vi "Scripting_G1DeleteToG3Delete.vi"(0 "VI Refnum":refnum<vi>, 1 "SearchVI":path=path "C:/classes/MainVI/MyGoop2/utils/MyGoop2_New.vi", 2 "Get":path=path "C:/classes/MainVI/MyGoop2/utils/MyGoop2_GetAttributesToModify.vi", 5 "error IO":errorcluster) -> (19 "error out":errorcluster)   [LabVIEW 2014]
uses:
  <vilib>/Utility/miscctls.llb/LVPositionTypeDef.ctl
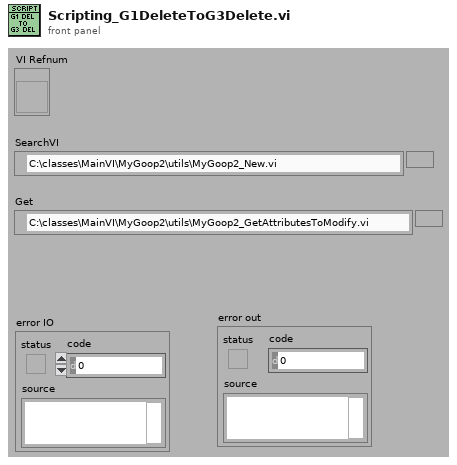
[diagram p1: front panel]
types:
  T1 = cluster{"Delete":refnum<vi>, "GetRef":refnum<vi>, "Block Diagram":refnum<vi>, "MergerErrors":refnum<vi>}
  T2 = typedef "LVPositionTypeDef.ctl" = cluster{"Left":i32, "Top":i32}
  T3 = typedef "LVRectTypeDef.ctl" = cluster{"Left":i16, "Top":i16, "Right":i16, "Bottom":i16}
  T4 = enum16{"Invalid Wire Rule", "Required", "Recommended", "Optional", "Dynamic Dispatch"}
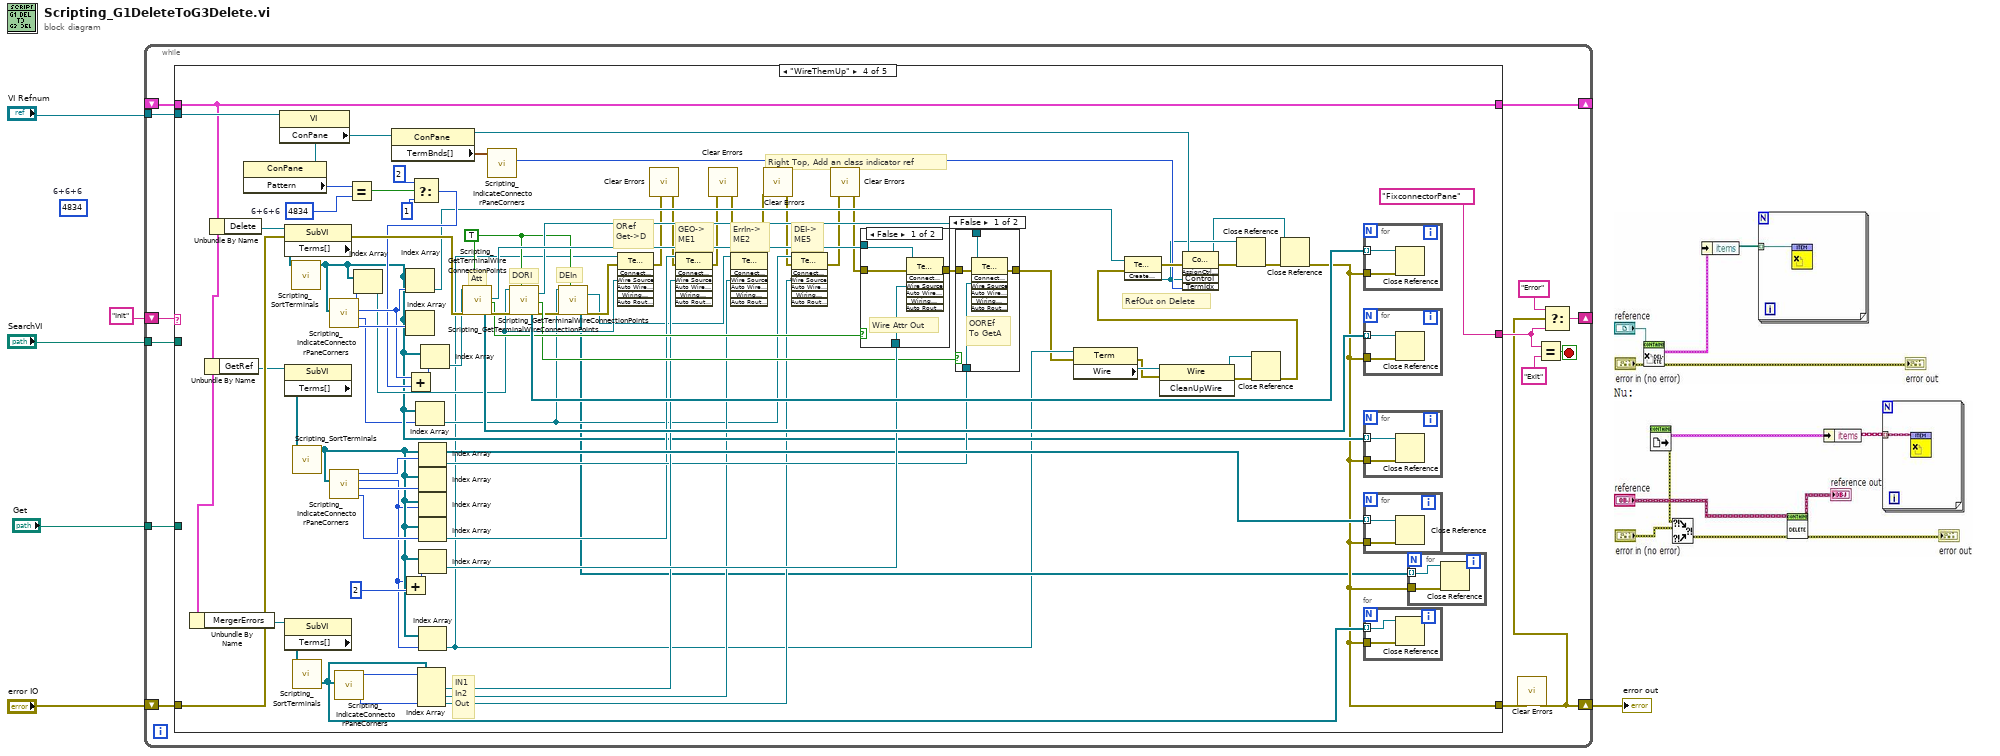
[diagram p0: block diagram]
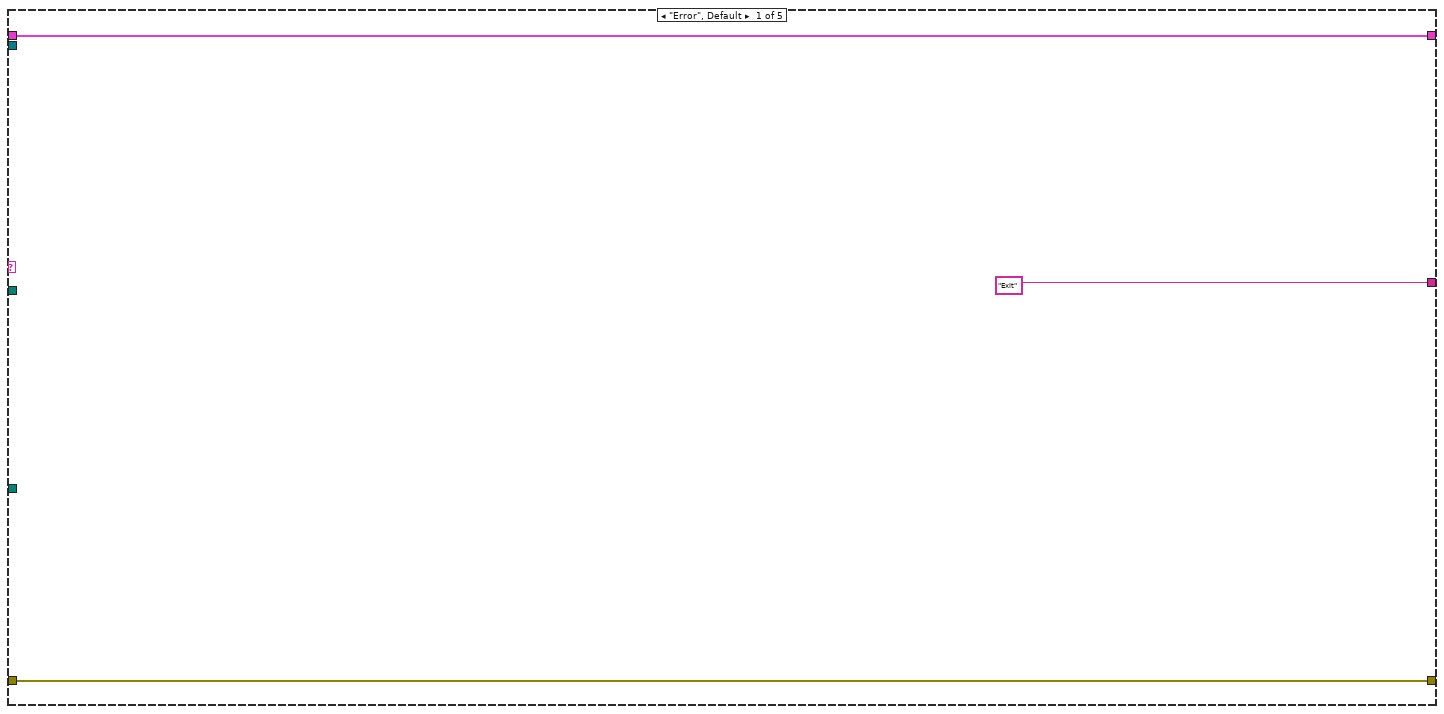
[diagram p2: hidden frame]
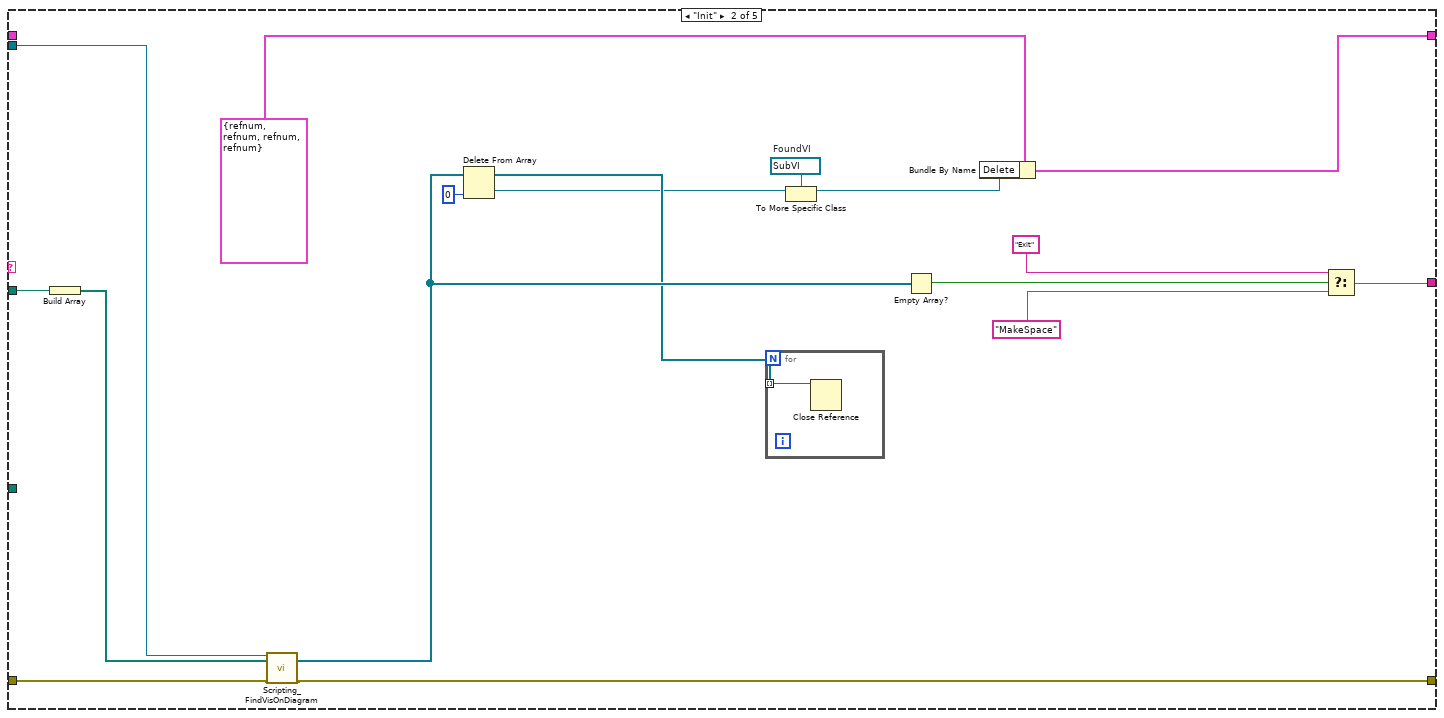
[diagram p3: hidden frame]
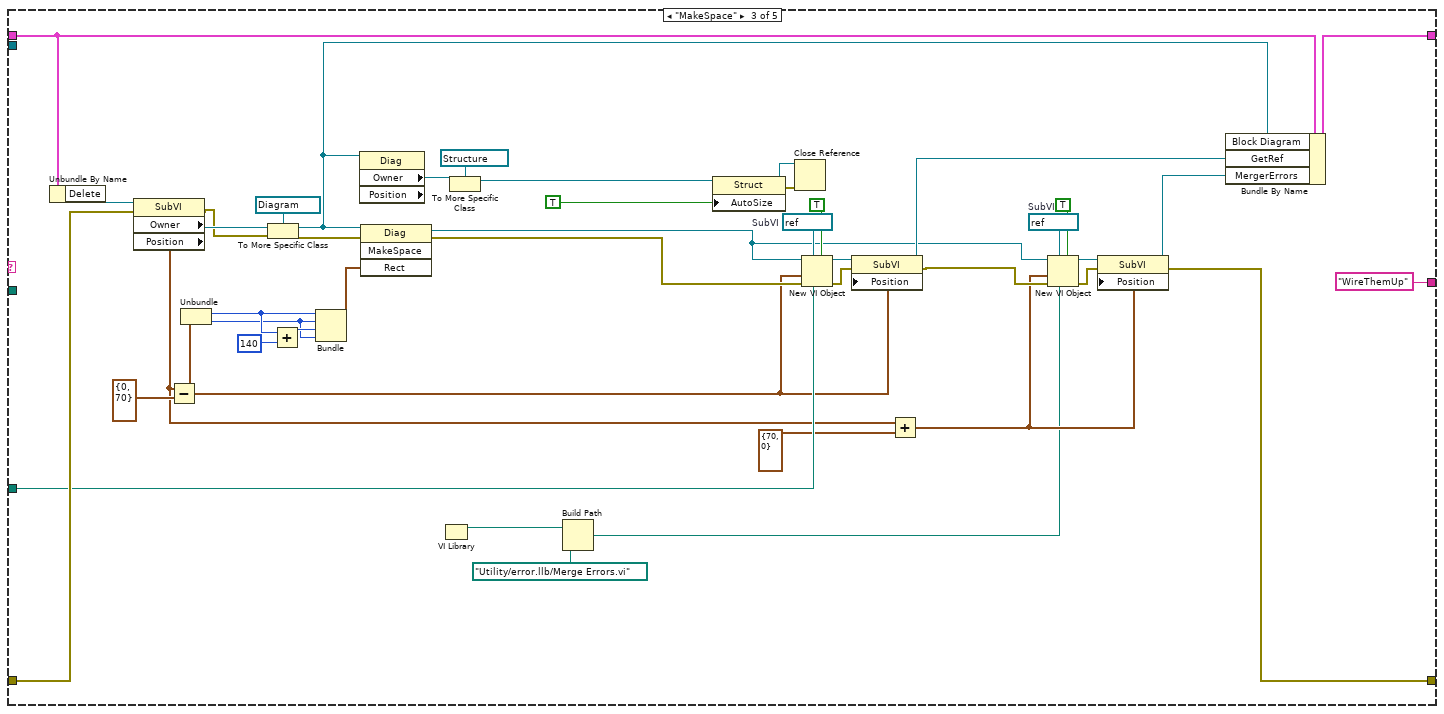
[diagram p4: hidden frame]
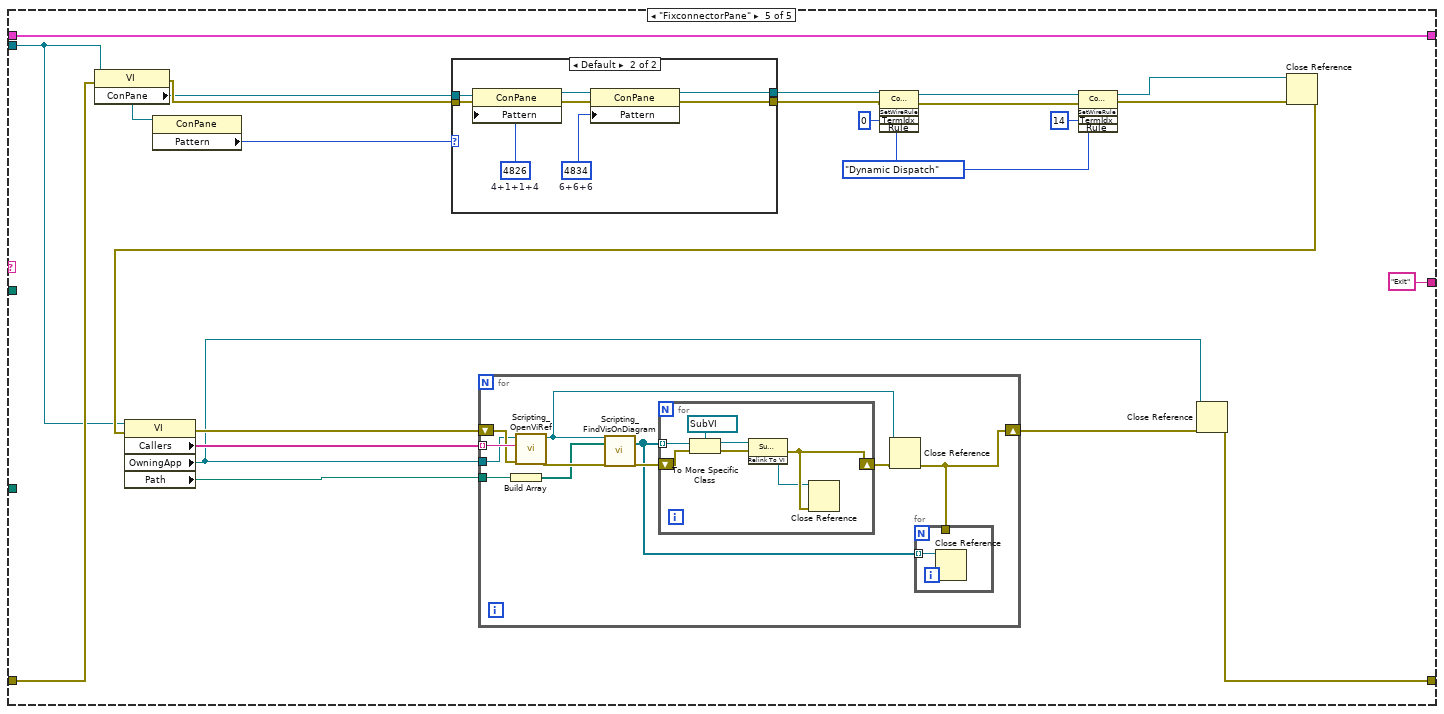
[diagram p7: hidden frame]
diagram:
  (unwired) u32 4834  # 6+6+6
  n1 = while {
    shift-right: [w7] -> w4
    shift-left: "error IO" -> [w20]
    shift-right: [w18] -> _
    shift-left: "Init" -> [w19]
    shift-right: [w13] -> _
    shift-left: _ -> [w12]
    tunnel: "VI Refnum" -> [w11]
    tunnel: "SearchVI" -> [w10]
    tunnel: "Get" -> [w9]
    stop <- w17 stop-if-true
    n2 = case shown="\"WireThemUp\"" w19 {
      tunnel: w20 -> [w23 w38 w84 w165 w210]
      tunnel: [w23 w37 w51 w102 w200] -> w8
      tunnel: ["Exit" w32 "WireThemUp" "FixconnectorPane" "Exit"] -> w14
      tunnel: [w21 w39 w62 w120 w209] -> w13
      tunnel: w12 -> [w21 _ w63 w120 w209]
      tunnel: w11 -> [_ w36 _ w132 w201]
      tunnel: w10 -> [_ w29 _ _ _]
      tunnel: w9 -> [_ _ w77 _ _]
      frame "Error", Default {
      }
      frame "Init" {
        w25 = refnum<vi> refnum  # FoundVI
        n3 = Build Array(w29) -> (w28:path[])
        n4 = call <resource>:"Scripting_FindVisOnDiagram.vi"("ViRef"=w36, "VIsToSerachFor/ViName"=w28, "error in (no error)"=w38) -> ("VisFound"=w31:refnum<vi>[], "error out"=w37:errorcluster)  [unwired: 15 in]
        n5 = Delete From Array(array=w31, index=0) -> (deleted portion=w26:refnum<vi>, array with subset deleted=w27:refnum<vi>[])  [unwired: 1 in]
        n6 = for {
          tunnel: w27 -> [w41] mode=indexing
          n7 = Close Reference(reference=w41) -> ()  [unwired: 1 in, 1 out]
        }
        n8 = To More Specific Class(target class=w25, reference=w26) -> (specific class reference=w24:refnum<vi>)  [unwired: 1 in, 1 out]
        n9 = Empty Array?(array=w31) -> (empty?=w35:bool)
        n10 = Bundle By Name(cluster=T1 {"Delete"=refnum, "GetRef"=refnum, "Block Diagram"=refnum, "MergerErrors"=refnum}, "Delete"=w24) -> (w39:T1)
        n11 = Select(t="Exit", s=w35, f="MakeSpace") -> (s? t:f=w32:string)
      }
      frame "MakeSpace" {
        w53 = refnum<vi> refnum  # SubVI
        w80 = refnum<vi> refnum  # SubVI
        n12 = Unbundle By Name(w63) -> ("Delete"=w85:refnum<vi>)
        n13 = property class="SubVI"(reference=w85, error in=w84) -> (error out=w81:errorcluster, "Owner"=w82:refnum<vi>, "Position"=w42:T2)  [unwired: 1 out]
        n14 = Subtract(x=w42, y=T2 {"Left"=0, "Top"=70}) -> (x-y=w50:T2)
        n15 = Unbundle(w50) -> ("Left"=w73:i32, "Top"=w70:i32)
        n16 = To More Specific Class(target class=refnum<vi> refnum ("Block Diagram"), reference=w82, error in=w81) -> (specific class reference=w58:refnum<vi>, error out=w67:errorcluster)
        n17 = Add(x=w73, y=i16 140 ("Right")) -> (x+y=w71:i32)
        n18 = Bundle("Left"=w73, "Top"=w70, w71, "Top"=w70) -> (w69:cluster{"Left":i32, "Top":i32, i32, "Top":i32})  [unwired: 1 in]
        n19 = property class="Diag" props=["Owner", "Position"](reference=w58) -> ("Owner"=w66:refnum<vi>)  [unwired: 1 in, 3 out]
        n20 = invoke class="Diag" method="MakeSpace"(reference=w58, error in=w67, "Rect"=w69) -> (reference out=w47:refnum<vi>, error out=w78:errorcluster)  [unwired: 1 in, 2 out]
        n21 = VI Library() -> (path=w57:path)
        n22 = To More Specific Class(target class=refnum<vi> refnum ("Block Diagram"), reference=w66) -> (specific class reference=w65:refnum<vi>)  [unwired: 1 in, 1 out]
        n23 = Build Path(base path=w57, name or relative path=path "Utility/error.llb/Merge Errors.vi") -> (appended path=w44:path)
        n24 = property class="Struct"(reference=w65, "AutoSize"=TRUE ("AutoSize To Fit Contents?")) -> (reference out=w59:refnum<vi>, error out=w60:errorcluster)  [unwired: 1 in]
        n25 = Close Reference(reference=w59, error in (no error)=w60) -> ()  [unwired: 1 out]
        n26 = New VI Object(vi object class=w80, auto wire? (F)=TRUE, owner refnum=w47, position/next to=w50, 6:w77, 8:w78) -> (object refnum=w76:refnum<vi>, 0:w75:errorcluster)  [unwired: 2 in]
        n27 = property class="SubVI"(reference=w76, error in=w75, "Position"=w50) -> (reference out=w61:refnum<vi>, error out=w52:errorcluster)
        n28 = Add(x=w42, y=T2 {"Left"=70, "Top"=0}) -> (x+y=w45:T2)
        n29 = New VI Object(vi object class=w53, auto wire? (F)=TRUE, owner refnum=w47, position/next to=w45, 6:w44, 8:w52) -> (object refnum=w55:refnum<vi>, 0:w56:errorcluster)  [unwired: 2 in]
        n30 = property class="SubVI"(reference=w55, error in=w56, "Position"=w45) -> (reference out=w46:refnum<vi>, error out=w51:errorcluster)
        n31 = Bundle By Name(cluster=w63, "Block Diagram"=w58, "GetRef"=w61, "MergerErrors"=w46) -> (w62:T1)
      }
      frame "WireThemUp" {
        w130 = u32 4834  # 6+6+6
        w111 = TRUE ("RemoveWire(Ture)")
        # "DEI->\nME5"
        # "DEIn"
        # "ErrIn->\nME2"
        # "ORef\nGet->D"
        # "GEO->\nME1"
        # "DORI"
        # "Att"
        # "RefOut on Delete"
        # "IN1\nIn2\nOut"
        # "Right Top, Add an class indicator ref"
        n32 = Unbundle By Name(w120) -> ("MergerErrors"=w121:refnum<vi>)
        n33 = Unbundle By Name(w120) -> ("GetRef"=w161:refnum<vi>)
        n34 = Unbundle By Name(w120) -> ("Delete"=w166:refnum<vi>)
        n35 = property class="VI"(reference=w132) -> ("ConPane"=w133:refnum<vi>)  [unwired: 1 in, 2 out]
        n36 = property class="ConPane"(reference=w133) -> ("Pattern"=w131:u32)  [unwired: 1 in, 2 out]
        n37 = property class="SubVI"(reference=w166, error in=w165) -> (error out=w164:errorcluster, "Terms[]"=w124:refnum<vi>[])  [unwired: 1 out]
        n38 = property class="SubVI"(reference=w161) -> ("Terms[]"=w150:refnum<vi>[])  [unwired: 1 in, 2 out]
        n39 = property class="SubVI"(reference=w121) -> ("Terms[]"=w122:refnum<vi>[])  [unwired: 1 in, 2 out]
        n40 = call <resource>:"Scripting_SortTerminals.vi"("Terminals[]"=w124) -> ("TerminalsOut[]"=w108:refnum<vi>[])  [unwired: 8 in, 2 out]
        n41 = call <resource>:"Scripting_SortTerminals.vi"("Terminals[]"=w150) -> ("TerminalsOut[]"=w145:refnum<vi>[])  [unwired: 8 in, 2 out]
        n42 = call <resource>:"Scripting_SortTerminals.vi"("Terminals[]"=w122) -> ("TerminalsOut[]"=w117:refnum<vi>[])  [unwired: 8 in, 2 out]
        n43 = call <resource>:"Scripting_IndicateConnectorPaneCorners.vi"("Terminals[]"=w108) -> ("RightLower"=w162:i32, "LeftLower"=w107:i32, "RightTop"=w135:i32, "LeftTop"=w123:i32)  [unwired: 7 in]
        n44 = call <resource>:"Scripting_IndicateConnectorPaneCorners.vi"("Terminals[]"=w145) -> ("RightLower"=w158:i32, "LeftLower"=w159:i32, "RightTop"=w144:i32, "LeftTop"=w160:i32)  [unwired: 7 in]
        n45 = call <resource>:"Scripting_IndicateConnectorPaneCorners.vi"("Terminals[]"=w117) -> ("RightLower"=w118:i32, "LeftTop"=w119:i32)  [unwired: 7 in, 2 out]
        n46 = Equal?(x=w131, y=w130) -> (x = y?=w129:bool)
        n47 = Index Array(array=w108, index=w123) -> (element=w116:refnum<vi>)
        n48 = property class="ConPane"(reference=w133) -> (reference out=w141:refnum<vi>, "TermBnds[]"=w143:T3[])  [unwired: 1 in, 1 out]
        n49 = Add(x=w144, y=2) -> (x+y=w149:i32)
        n50 = Index Array(array=w108, index=w135) -> (element=w125:refnum<vi>)
        n51 = Index Array(array=w108, index=w162) -> ()  [unwired: 1 out]
        n52 = Select(t=2 ("y"), s=w129, f=1) -> (s? t:f=w128:i32)
        n53 = Add(x=w135, y=w128) -> (x+y=w134:i32)
        n54 = Index Array(array=w108, index=w107) -> (element=w104:refnum<vi>)
        n55 = Index Array(array=w117, index #1=w119, index #3=w118) -> (element #1=w114:refnum<vi>, element #2=w105:refnum<vi>, element #3=w103:refnum<vi>)  [unwired: 1 in]
        n56 = Index Array(array=w145, index=w160) -> (element=w110:refnum<vi>)
        n57 = Index Array(array=w145, index=w159) -> ()  [unwired: 1 out]
        n58 = Index Array(array=w145, index=w144) -> ()  [unwired: 1 out]
        n59 = Index Array(array=w145, index=w158) -> (element=w109:refnum<vi>)
        n60 = Index Array(array=w145, index=w149) -> (element=w148:refnum<vi>)
        n61 = Index Array(array=w145, index=w144) -> (element=w98:refnum<vi>)
        n62 = Index Array(array=w108, index=w134) -> (element=w152:refnum<vi>)
        n63 = call <resource>:"Scripting_GetTerminalWireConnectionPoints.vi"("Term Refnum In"=w152, "error in"=w164, "RemoveWire(False)"=w111) -> ("AllWireTerminals"=w154:refnum<vi>[], "FirstWireTermDrain"=w157:refnum<vi>, "NoWireConnected"=w147:bool, "error out"=w163:errorcluster)  [unwired: 8 in, 5 out]
        n64 = call <resource>:"Scripting_IndicateConnectorPaneCorners.vi"("TermBnds[]"=w143) -> ("RightTop"=w140:i32)  [unwired: 7 in, 3 out]
        n65 = call <resource>:"Scripting_GetTerminalWireConnectionPoints.vi"("Term Refnum In"=w116, "error in"=w163, "RemoveWire(False)"=w111) -> ("AllWireTerminals"=w155:refnum<vi>[], "WireTermSource"=w115:refnum<vi>, "NoWireConnected"=w146:bool, "error out"=w113:errorcluster)  [unwired: 8 in, 5 out]
        n66 = call <resource>:"Scripting_GetTerminalWireConnectionPoints.vi"("Term Refnum In"=w104, "error in"=w113, "RemoveWire(False)"=w111) -> ("AllWireTerminals"=w101:refnum<vi>[], "WireTermSource"=w106:refnum<vi>, "error out"=w112:errorcluster)  [unwired: 8 in, 6 out]
        n67 = invoke class="Term" method="Connect Wire"(reference=w98, error in=w112, "Wire Source"=w116) -> (error out=w93:errorcluster)  [unwired: 4 in, 6 out]
        n68 = call <vilib>:"Clear Errors.vi"("error in (no error)"=w93) -> ("error out"=w92:errorcluster)  [unwired: 5 in, 1 out]
        n69 = invoke class="Term" method="Connect Wire"(reference=w109, error in=w92, "Wire Source"=w114) -> (error out=w91:errorcluster)  [unwired: 4 in, 6 out]
        n70 = call <vilib>:"Clear Errors.vi"("error in (no error)"=w91) -> ("error out"=w90:errorcluster)  [unwired: 5 in, 1 out]
        n71 = invoke class="Term" method="Connect Wire"(reference=w106, error in=w90, "Wire Source"=w105) -> (error out=w89:errorcluster)  [unwired: 4 in, 6 out]
        n72 = call <vilib>:"Clear Errors.vi"("error in (no error)"=w89) -> ("error out"=w88:errorcluster)  [unwired: 5 in, 1 out]
        n73 = invoke class="Term" method="Connect Wire"(reference=w104, error in=w88, "Wire Source"=w103) -> (error out=w87:errorcluster)  [unwired: 4 in, 6 out]
        n74 = call <vilib>:"Clear Errors.vi"("error in (no error)"=w87) -> ("error out"=w86:errorcluster)  [unwired: 5 in, 1 out]
        n75 = case shown="False" w147 {
          tunnel: w157 -> [w179 _]
          tunnel: [w178 w180] -> w156
          tunnel: w86 -> [w177 w180]
          tunnel: w148 -> [w176 _]
          frame False {
            # "Wire Attr Out"
            n76 = invoke class="Term" method="Connect Wire"(reference=w179, error in=w177, "Wire Source"=w176) -> (error out=w178:errorcluster)  [unwired: 4 in, 6 out]
          }
          frame True {
          }
        }
        n77 = case shown="False" w146 {
          tunnel: w115 -> [w174 _]
          tunnel: w156 -> [w173 w175]
          tunnel: [w172 w175] -> w94
          tunnel: w110 -> [w171 _]
          frame False {
            # "OOREf\nTo GetA"
            n78 = invoke class="Term" method="Connect Wire"(reference=w174, error in=w173, "Wire Source"=w171) -> (error out=w172:errorcluster)  [unwired: 4 in, 6 out]
          }
          frame True {
          }
        }
        n79 = property class="Term"(reference=w98, error in=w94) -> (error out=w99:errorcluster, "Wire"=w100:refnum<vi>)  [unwired: 1 out]
        n80 = invoke class="Wire" method="CleanUpWire"(reference=w100, error in=w99) -> (reference out=w96:refnum<vi>, error out=w97:errorcluster)  [unwired: 1 in, 1 out]
        n81 = Close Reference(reference=w96, error in (no error)=w97) -> (error out=w95:errorcluster)
        n82 = invoke class="Term" method="Create Indicator"(reference=w125, error in=w95) -> (error out=w142:errorcluster, "Create Indicator"=w138:refnum<vi>)  [unwired: 1 in, 1 out]
        n83 = invoke class="ConPane" method="AssignCtrlToTerm"(reference=w141, error in=w142, "Control"=w138, "TermIdx"=w140) -> (reference out=w136:refnum<vi>, error out=w139:errorcluster)  [unwired: 1 in, 3 out]
        n84 = Close Reference(reference=w138, error in (no error)=w139) -> (error out=w137:errorcluster)
        n85 = Close Reference(reference=w136, error in (no error)=w137) -> (error out=w102:errorcluster)
        n86 = for {
          tunnel: w102 -> [w188]
          tunnel: w155 -> [w187] mode=indexing
          n87 = Close Reference(reference=w187, error in (no error)=w188) -> ()  [unwired: 1 out]
        }
        n88 = for {
          tunnel: w102 -> [w186]
          tunnel: w154 -> [w185] mode=indexing
          n89 = Close Reference(reference=w185, error in (no error)=w186) -> ()  [unwired: 1 out]
        }
        n90 = for {
          tunnel: w102 -> [w184]
          tunnel: w108 -> [w183] mode=indexing
          n91 = Close Reference(reference=w183, error in (no error)=w184) -> ()  [unwired: 1 out]
        }
        n92 = for {
          tunnel: w102 -> [w182]
          tunnel: w145 -> [w181] mode=indexing
          n93 = Close Reference(reference=w181, error in (no error)=w182) -> ()  [unwired: 1 out]
        }
        n94 = for {
          tunnel: w102 -> [w170]
          tunnel: w117 -> [w169] mode=indexing
          n95 = Close Reference(reference=w169, error in (no error)=w170) -> ()  [unwired: 1 out]
        }
        n96 = for {
          tunnel: w102 -> [w168]
          tunnel: w101 -> [w167] mode=indexing
          n97 = Close Reference(reference=w167, error in (no error)=w168) -> ()  [unwired: 1 out]
        }
      }
      frame "FixconnectorPane" {
        w191 = T4."Dynamic Dispatch" ("Rule")
        n98 = property class="VI"(reference=w201, error in=w210) -> (error out=w211:errorcluster, "ConPane"=w190:refnum<vi>)  [unwired: 1 out]
        n99 = property class="ConPane"(reference=w190) -> ("Pattern"=w189:u32)  [unwired: 1 in, 2 out]
        n100 = case shown="Default" w189 {
          tunnel: w211 -> [w212 w221]
          tunnel: [w213 w216] -> w199
          tunnel: [w212 w215] -> w197
          tunnel: w190 -> [w213 w214]
          frame 4834 {
          }
          frame Default {
            w220 = u32 4826  # 4+1+1+4
            w217 = u32 4834  # 6+6+6
            n101 = property class="ConPane"(reference=w214, error in=w221, "Pattern"=w220) -> (reference out=w219:refnum<vi>, error out=w218:errorcluster)
            n102 = property class="ConPane"(reference=w219, error in=w218, "Pattern"=w217) -> (reference out=w216:refnum<vi>, error out=w215:errorcluster)
          }
        }
        n103 = invoke class="ConPane" method="SetWireRule"(reference=w199, error in=w197, "TermIdx"=u32 0 ("Terminal Index"), "Rule"=w191) -> (reference out=w196:refnum<vi>, error out=w195:errorcluster)  [unwired: 1 in, 3 out]
        n104 = invoke class="ConPane" method="SetWireRule"(reference=w196, error in=w195, "TermIdx"=u32 14 ("Terminal Index"), "Rule"=w191) -> (reference out=w193:refnum<vi>, error out=w192:errorcluster)  [unwired: 1 in, 3 out]
        n105 = Close Reference(reference=w193, error in (no error)=w192) -> (error out=w202:errorcluster)
        n106 = property class="VI"(reference=w201, error in=w202) -> (error out=w206:errorcluster, "Callers"=w207:string[], "OwningApp"=w203:refnum<vi>, "Path"=w205:path)  [unwired: 1 out]
        n107 = for {
          tunnel: w207 -> [w232] mode=indexing
          tunnel: w205 -> [w229]
          tunnel: w203 -> [w225]
          shift-right: [w222] -> w204
          shift-left: w206 -> [w231]
          n108 = Build Array(w229) -> (w228:path[])
          n109 = call <resource>:"Scripting_OpenViRef.vi"("error in"=w231, "ViPath/ViName/Viref"=w232, "AppRef"=w225) -> ("error out"=w230:errorcluster, "vi reference"=w223:refnum<vi>)  [unwired: 6 in, 1 out]
          n110 = call <resource>:"Scripting_FindVisOnDiagram.vi"("ViRef"=w223, "VIsToSerachFor/ViName"=w228, "error in (no error)"=w230) -> ("VisFound"=w226:refnum<vi>[], "error out"=w227:errorcluster)  [unwired: 15 in]
          n111 = for {
            tunnel: w226 -> [w239] mode=indexing
            shift-right: [w235] -> w224
            shift-left: w227 -> [w238]
            n112 = To More Specific Class(target class=refnum<vi> refnum ("WhileLoop"), reference=w239, error in=w238) -> (specific class reference=w237:refnum<vi>, error out=w236:errorcluster)
            n113 = invoke class="SubVI" method="Relink To VI"(reference=w237, error in=w236) -> (error out=w235:errorcluster, "Relink To VI"=w234:refnum<vi>)  [unwired: 1 in, 1 out]
            n114 = Close Reference(reference=w234, error in (no error)=w235) -> ()  [unwired: 1 out]
          }
          n115 = Close Reference(reference=w223, error in (no error)=w224) -> (error out=w222:errorcluster)
          n116 = for {
            tunnel: w226 -> [w233] mode=indexing
            tunnel: w222 -> [_]
            n117 = Close Reference(reference=w233) -> ()  [unwired: 1 in, 1 out]
          }
        }
        n118 = Close Reference(reference=w203, error in (no error)=w204) -> (error out=w200:errorcluster)
      }
    }
    n119 = call <vilib>:"Clear Errors.vi"("error in (no error)"=w8) -> ("error out"=w7:errorcluster)  [unwired: 5 in, 1 out]
    n120 = Equal?(x=w14, y="Exit") -> (x = y?=w17:bool)
    n121 = Select(t="Error", s=w7, f=w14) -> (s? t:f=w18:string)
  }
  "error out" <- w4
